vi "StartTopicServer.vi"(0 "Server Direction":enum16{"Start Server", "Close Server"}(ring), 2 "ROS in":T1={"topic port"=0, "Node"="", "topic"="", "type"="", "node port"=0, "error "={"status"=FALSE, "code"=0, "source"=""}, "Direction"=enum."Node", "APIs"=[], "Update (ms)"=1, "write queue"=1}, 3 "Priority":enum16{"In Front", "In Back"}(ring)=enum."In Back") -> (4 "ROS out":T1={"topic port"=0, "Node"="", "topic"="", "type"="", "node port"=0, "error "={"status"=FALSE, "code"=0, "source"=""}, "Direction"=enum."Node", "APIs"=[], "Update (ms)"=1, "write queue"=1})   [LabVIEW 2010]
uses:
  _ROSDirection.ctl
  _ROSControl.ctl
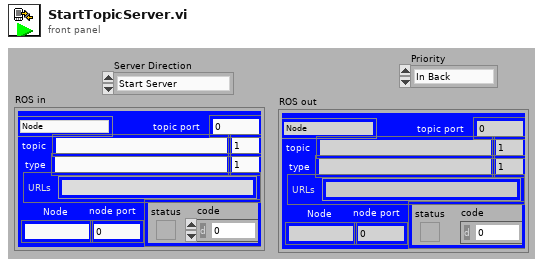
[diagram p1: front panel]
types:
  T1 = typedef "_ROSControl.ctl" = cluster{"topic port":u16, "Node":string, "topic":string, "type":string, "node port":u32, "error ":errorcluster, "Direction":T2, "APIs":string[], "Update (ms)":u16, "write queue":u16}
  T2 = typedef "_ROSDirection.ctl" = enum16{"Node", "Publisher", "Subscriber", "Service Client"}
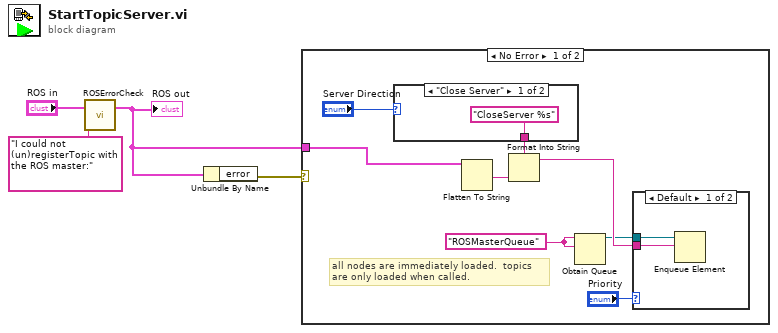
[diagram p0: block diagram]
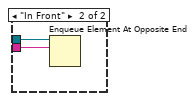
[diagram p2: hidden frame]
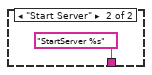
[diagram p3: hidden frame]
diagram:
  n1 = call "ROSErrorCheck.vi"("message"="I could not (un)registerTopic with the ROS master:", "ROS in"="ROS in") -> ("ROS out"=w1:T1)  [unwired: 1 in]
  "ROS out" <- w1
  n2 = Unbundle By Name(w1) -> ("error"=w4:errorcluster)
  n3 = case shown="No Error" w4 {
    tunnel: w1 -> [w7 _]
    frame No Error {
      w8 = "ROSMasterQueue" ("name (unnamed)")
      # "all nodes are immediately loaded.  topics\nare only loaded when called."
      n4 = case shown="\"Close Server\"" "Server Direction" {
        tunnel: ["CloseServer %s" ("format string") "StartServer %s" ("format string")] -> w11
        frame "Close Server" {
        }
        frame "Start Server" {
        }
      }
      n5 = Flatten To String(anything=w7) -> (data string=w6:string)  [unwired: 3 in, 2 out]
      n6 = Format Into String(format string=w11, w6) -> (resulting string=w10:string)  [unwired: 2 in, 1 out]
      n7 = Obtain Queue(name (unnamed)=w8, element data type=w8) -> (queue out=w9:refnum<queue>)  [unwired: 3 in, 2 out]
      n8 = case shown="Default" "Priority" {
        tunnel: w10 -> [w13 w16]
        tunnel: w9 -> [w14 w15]
        frame Default {
          n9 = Enqueue Element(queue=w14, element=w13) -> ()  [unwired: 2 in, 3 out]
        }
        frame "In Front" {
          n10 = Enqueue Element At Opposite End(queue=w15, element=w16) -> ()  [unwired: 2 in, 3 out]
        }
      }
    }
    frame Error {
    }
  }
